vi "MakeWall.vi"(8 "error in (no error)":errorcluster, 11 "MazeGame in":refnum<class "MazeGame.lvclass">) -> (0 "error out":errorcluster, 2 "Wall":refnum<class "Wall.lvclass">, 3 "MazeGame out":refnum<class "MazeGame.lvclass">)   [LabVIEW 2020, in "FactoryMethod.lvlib" / "NoParametrizedFactoryMethod.lvlib" / "MazeGame.lvclass"]
uses:
  MazeGame.lvclass
  GoFcommonClasses/ConcreteMazeSite/Wall/Wall.lvclass
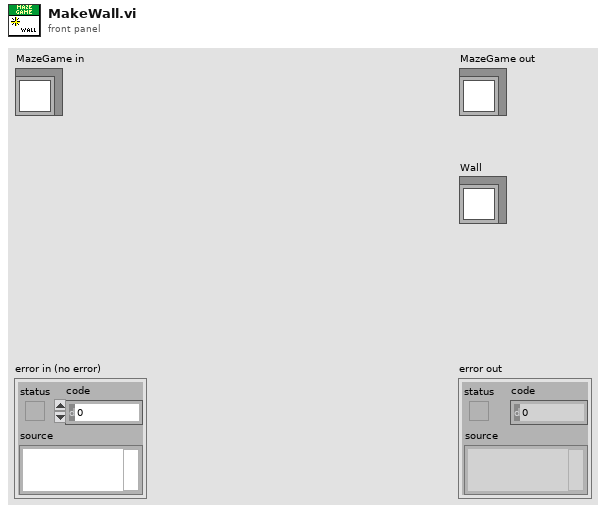
[diagram p1: front panel]
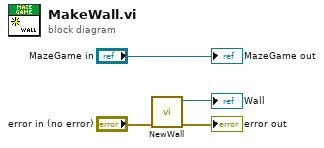
[diagram p0: block diagram]
diagram:
  n1 = call "NewWall.vi"("error in (no error)"="error in (no error)") -> ("error out"=→"error out":errorcluster, "Wall"=→"Wall":refnum<class "Wall.lvclass">)  [unwired: 9 in]
  "MazeGame out" <- "MazeGame in"
